vi "Print Diploma.vi"(7 "Length Diploma":string, 8 "error in (no error)":errorcluster, 9 "Name":string, 10 "Printer Name":string, 11 "Diploma Template Path":path) -> (0 "error out":errorcluster)   [LabVIEW 2018]
uses:
  <vilib>/Utility/NIReport.llb/Report Type.ctl
  <vilib>/addons/_office/word.llb/Word Find & Replace (str).vi
  <vilib>/Utility/NIReport.llb/NI_report.lvclass
  <vilib>/addons/_office/NI_ReportGenerationToolkit.lvlib
  <vilib>/Utility/NIReport.llb/Word/NI_Word.lvclass
  <vilib>/Utility/NIReport.llb/NI_ReportGenerationCore.lvlib
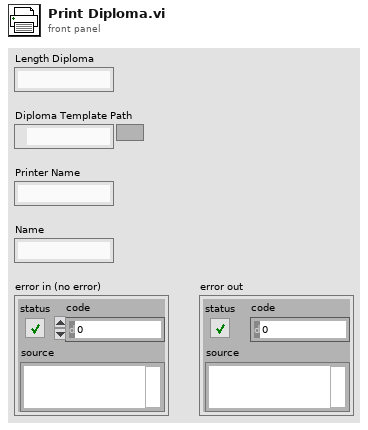
[diagram p1: front panel]
types:
  T1 = typedef "NI_ReportGenerationCore.lvlib/Report Type.ctl" = enum16{"HTML", "Word", "Excel"}
  T2 = enum16{"maximized", "minimized", "normal", "no change"}
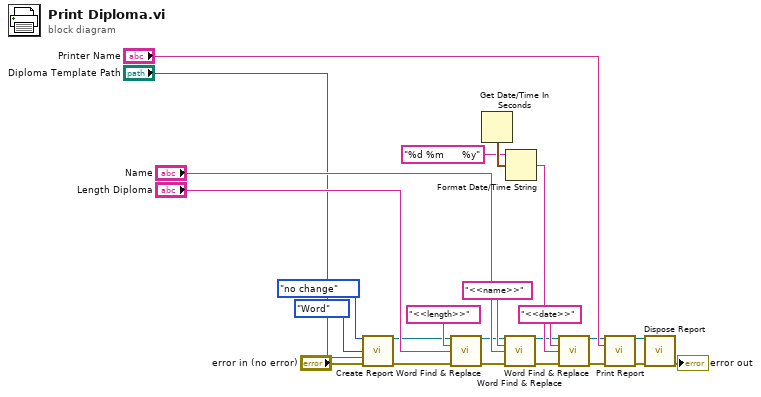
[diagram p0: block diagram]
diagram:
  n1 = call <vilib>:"Create Report.vi"("window state (normal)"=T2."no change", "report type"=Report_Type."Word", "template (empty)"="Diploma Template Path", "error in (no error)"="error in (no error)") -> ("report out"=w4:refnum<class "NI_report.lvclass">, "error out"=w1:errorcluster)  [unwired: 10 in]
  n2 = call-poly <vilib>:"Word Find & Replace.vi"("report in"=w4, "find what?"="<<length>>", "replace with"="Length Diploma", "error in (no error)"=w1) -> ("report out"=w5:refnum<class "NI_report.lvclass">, "error out"=w2:errorcluster)  [unwired: 9 in, 1 out]
  n3 = Get Date/Time In Seconds() -> (seconds since 1Jan1904=w17:timestamp)
  n4 = call-poly <vilib>:"Word Find & Replace.vi"("report in"=w5, "find what?"="<<name>>", "replace with"="Name", "error in (no error)"=w2) -> ("report out"=w6:refnum<class "NI_report.lvclass">, "error out"=w3:errorcluster)  [unwired: 9 in, 1 out]
  n5 = Format Date/Time String(time format string (%c)="%d %m      %y", seconds (now)=w17) -> (date/time string=w18:string)  [unwired: 1 in]
  n6 = call-poly <vilib>:"Word Find & Replace.vi"("report in"=w6, "find what?"="<<date>>", "replace with"=w18, "error in (no error)"=w3) -> ("report out"=w13:refnum<class "NI_report.lvclass">, "error out"=w10:errorcluster)  [unwired: 9 in, 1 out]
  n7 = call-dynamic "Print Report.vi"("report in"=w13, "printer name (default)"="Printer Name", "error in (no error)"=w10) -> ("report out"=w12:refnum<class "NI_report.lvclass">, "error out"=w11:errorcluster)  [unwired: 11 in]
  n8 = call-dynamic "Dispose Report.vi"("report in"=w12, "error in (no error)"=w11) -> ("error out"=→"error out":errorcluster)  [unwired: 13 in]
